vi "lookup.vi"() -> (1 "确定":bool, 2 "选择器 2":T1(ring))   [LabVIEW 2018]
panel:
  in  "选择":T1(ring)
  in  "确定":bool
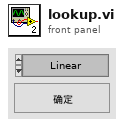
[diagram p1: front panel]
types:
  T1 = enum32{"Linear", "Log", "Exp", "Square", "Square root", "Power X", "Power 1/X"}
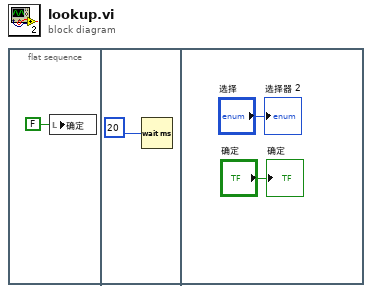
[diagram p0: block diagram]
diagram:
  n1 = flat-sequence {
    frame #0 {
      n2 = local write "确定"(FALSE ("确定")) -> ()
    }
    frame #1 {
      n3 = Wait (ms)(milliseconds to wait=u32 20 ("等待时间（毫秒）")) -> ()  [unwired: 1 out]
    }
    frame #2 {
      "确定" <- "确定"
      "选择器 2" <- "选择"
    }
  }
